vi "CurrentControl.vi"(0 "Current Control Parameters":T2, 7 "FPGA Data":T1, 11 "Error In":errorcluster) -> (4 "Current Out":dbl, 15 "Error Out":errorcluster)   [LabVIEW 2013]
uses:
  eng/trunk/ni/cRIO Master Files/Controls/CurrentControlParameters.ctl
  Controls/FPGAData.ctl
  <vilib>/functionblocks/Control/PID/PID.vi
  <vilib>/functionblocks/FB Core/FB Core.xnode
  <vilib>/functionblocks/FB Property/FB Overlay DBL.ctl
  <vilib>/functionblocks/NI_FunctionBlock Libraries.lvlib
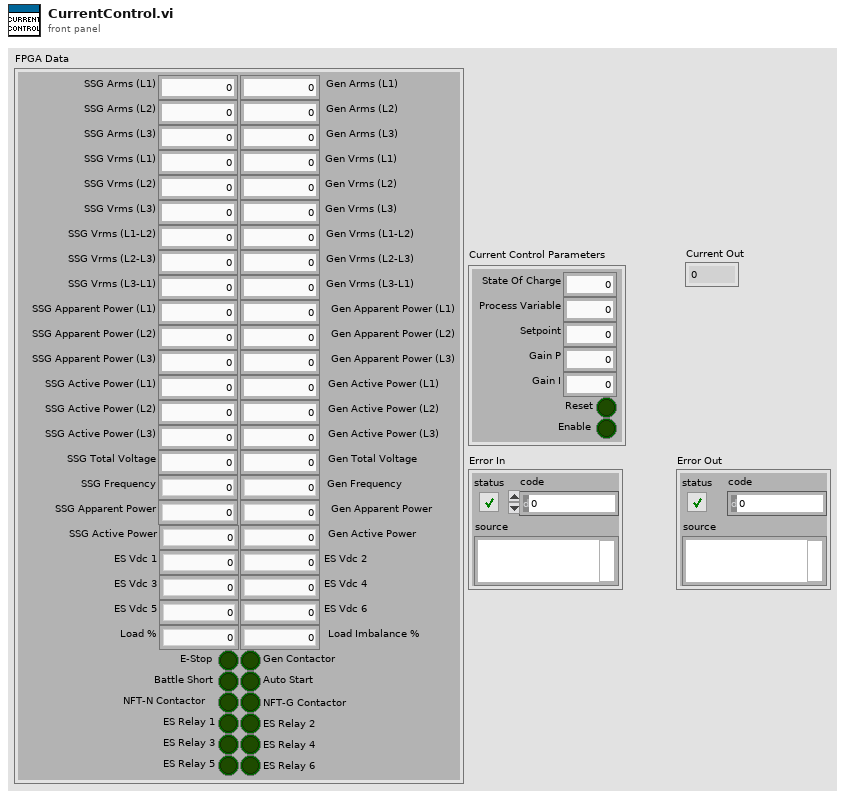
[diagram p1: front panel]
types:
  T1 = typedef "FPGAData.ctl" = cluster{"SSG Frequency":sgl, "SSG Total Voltage":dbl, "SSG Active Power":sgl, "SSG Apparent Power":sgl, "SSG Active Power (L1)":dbl, "SSG Active Power (L2)":dbl, "SSG Active Power (L3)":dbl, "SSG Apparent Power (L1)":dbl, "SSG Apparent Power (L2)":dbl, "SSG Apparent Power (L3)":dbl, "SSG Vrms (L1-L2)":dbl, "SSG Vrms (L2-L3)":dbl, "SSG Vrms (L3-L1)":dbl, "SSG Vrms (L1)":dbl, "SSG Vrms (L2)":dbl, "SSG Vrms (L3)":dbl, "SSG Arms (L1)":dbl, "SSG Arms (L2)":dbl, "SSG Arms (L3)":dbl, "Gen Frequency":sgl, "Gen Total Voltage":dbl, "Gen Active Power":sgl, "Gen Apparent Power":sgl, "Gen Active Power (L1)":dbl, "Gen Active Power (L2)":dbl, "Gen Active Power (L3)":dbl, "Gen Apparent Power (L1)":dbl, "Gen Apparent Power (L2)":dbl, "Gen Apparent Power (L3)":dbl, "Gen Vrms (L1-L2)":dbl, "Gen Vrms (L2-L3)":dbl, "Gen Vrms (L3-L1)":dbl, "Gen Vrms (L1)":dbl, "Gen Vrms (L2)":dbl, "Gen Vrms (L3)":dbl, "Gen Arms (L1)":dbl, "Gen Arms (L2)":dbl, "Gen Arms (L3)":dbl, "ES Vdc 1":sgl, "ES Vdc 2":sgl, "Load %":sgl, "Load Imbalance %":sgl, "E-Stop":bool, "Battle Short":bool, "Auto Start":bool, "Gen Contactor":bool, "ES Relay 1":bool, "ES Relay 2":bool, "NFT-N Contactor":bool, "NFT-G Contactor ":bool, "ES Relay 3":bool, "ES Relay 4":bool, "ES Relay 5":bool, "ES Relay 6":bool, "ES Vdc 3":sgl, "ES Vdc 4":sgl, "ES Vdc 5":sgl, "ES Vdc 6":sgl}
  T2 = typedef "CurrentControlParameters.ctl" = cluster{"State Of Charge":sgl, "Process Variable":dbl, "Setpoint":dbl, "Gain P":dbl, "Gain I":dbl, "Reset":bool, "Enable":bool}
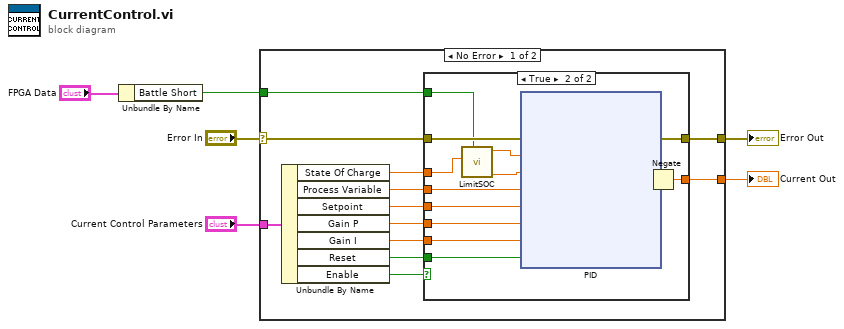
[diagram p0: block diagram]
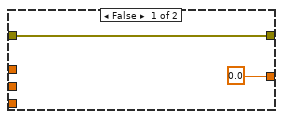
[diagram p2: hidden frame]
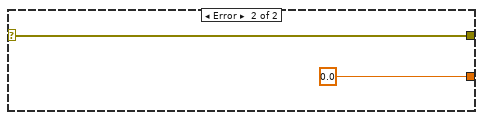
[diagram p3: hidden frame]
diagram:
  n1 = Unbundle By Name("FPGA Data") -> ("Battle Short"=w1:bool)
  n2 = case shown="No Error" "Error In" {
    selector: "Error In" -> [w16 w100]
    tunnel: [w18 w100] -> w4
    tunnel: [w17 0.0] -> w5
    tunnel: "Current Control Parameters" -> [w15 _]
    tunnel: w1 -> [w7 _]
    frame No Error {
      n3 = Unbundle By Name(w15) -> ("State Of Charge"=w8:sgl, "Process Variable"=w9:dbl, "Setpoint"=w10:dbl, "Gain P"=w11:dbl, "Gain I"=w12:dbl, "Reset"=w13:bool, "Enable"=w14:bool)
      n4 = case shown="True" w14 {
        tunnel: [w19 w33] -> w18
        tunnel: [0.0 w31] -> w17
        tunnel: w16 -> [w19 w28]
        tunnel: w13 -> [_ w27]
        tunnel: w12 -> [_ w26]
        tunnel: w11 -> [_ w25]
        tunnel: w10 -> [_ w24]
        tunnel: w9 -> [_ w23]
        tunnel: w8 -> [_ w22]
        tunnel: w7 -> [_ w21]
        frame False {
        }
        frame True {
          n5 = call "LimitSOC.vi"("Battle Short"=w21, "SOC Actual"=w22) -> ("Output Low"=w29:dbl, "Output High"=w30:dbl)  [unwired: 6 in]
          n6 = xnode "PID"("error in"=w28, "output high"=w30, "output low"=w29, "process variable"=w23, "setpoint"=w24, "proportional gain (Kc)"=w25, "integral time (Ti, min)"=w26, "reinitialize? (F)"=w27) -> ("error out"=w33:errorcluster, "output"=w32:dbl)
          n7 = Negate(x=w32) -> (-x=w31:dbl)
        }
      }
    }
    frame Error {
    }
  }
  "Current Out" <- w5
  "Error Out" <- w4
